vi "LCD Reader.vi"(6 "Retardance":dbl[unit]=8.32e-07, 7 "PEM in Exc. Mode?":bool, 8 "error in (no error)":errorcluster, 9 "LCD Retarder in":refnum<class "LCD Retarder.lvclass">, 10 "Reader.lvclass":refnum<class "Reader.lvclass">, 11 "LCD Reader in":refnum<class "LCD Reader.lvclass">) -> (0 "error out":errorcluster, 3 "LCD Reader out":refnum<class "LCD Reader.lvclass">)   [LabVIEW 2009, in "LCD Reader.lvclass"]
uses:
  LCD Reader.lvclass
  Reader/Reader.lvclass
  Instruments/LCD/LCD Retarder.lvclass
  LCD Reader.lvclass/LCD Reader.ctl
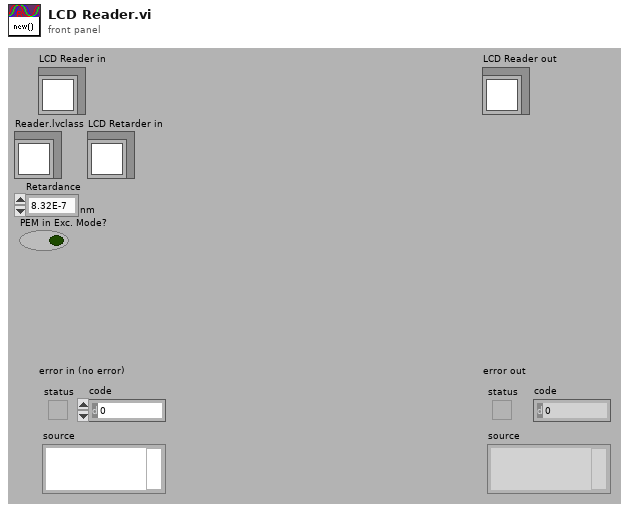
[diagram p1: front panel]
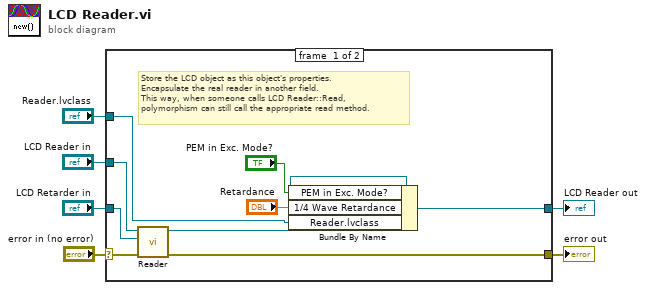
[diagram p0: block diagram]
diagram:
  n1 = case shown="No Error" "error in (no error)" {
    selector: "error in (no error)" -> [w12 w17]
    tunnel: [w11 w17] -> w5
    tunnel: [w15 w16] -> w3
    tunnel: "LCD Reader in" -> [w13 w16]
    tunnel: "Reader.lvclass" -> [w14 _]
    tunnel: "LCD Retarder in" -> [w10 _]
    frame #0 {
      # "Store the LCD object as this object's properties.\nEncapsulate the real reader in another field.\nThis way, when someone calls LCD Reader::Read,\npolymorphism can still call the appropriate read method."
      n2 = call "Reader.vi"("error in (no error)"=w12, "Readable"=w10, "Reader in"=w13) -> ("error out"=w11:errorcluster, "Reader out"=w9:refnum<class "LCD Reader.lvclass">)  [unwired: 7 out]
      n3 = Bundle By Name(cluster=w9, "PEM in Exc. Mode?"="PEM in Exc. Mode?", "1/4 Wave Retardance"="Retardance", "Reader.lvclass"=w14) -> (w15:refnum<class "LCD Reader.lvclass">)
    }
    frame #1 {
    }
  }
  "error out" <- w5
  "LCD Reader out" <- w3
